vi "ma_Tone estimation subroutine G(f) (FFT input) (CDB).vi"(8 "N (window length)":i32=512, 9 "window":u16(ring) items=["Rectangle"=0, "Hanning"=1, "Hamming"=2, "Blackman-Harris"=3, "Exact Blackman"=4, "Blackman"=5, "Flat Top"=6, "4 Term B-Harris "=7, "7 Term B-Harris"=8, "Low Sidelobe"=9, "Blackman Nuttall"=11, "Triangle"=30, "Bartlett-Hanning"=31, "Bohman"=32, "Parzen"=33, "Welch"=34, "Kaiser"=60, "Dolph-Chebyshev"=61, "Gaussian"=62], 10 "frequency":dbl format="%.5e", 11 "three fingers":T1={"f0"=0.0, "df"=1.0, "spectrum"=[]} {"spectrum" format="%.2f"; "df" format="%.2f"; "f0" format="%.2f"}) -> (1 "phase [degree]":dbl format="%.2f", 2 "Amplitude":dbl format="%.2f", 3 "G(f)":dbl format="%.2e")   [LabVIEW 2020, in "NI_MAPro.lvlib"]
uses:
  NI_MAPro.lvlib
  ma_sml_Spectrum Cluster (complex).ctl
  NI_AALBase.lvlib
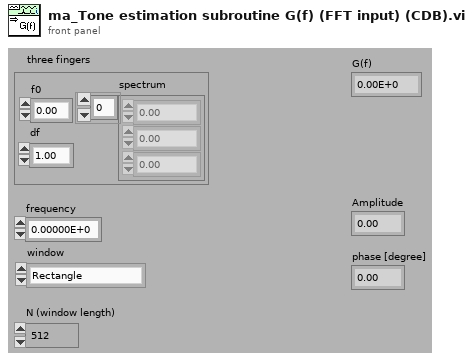
[diagram p1: front panel]
types:
  T1 = typedef "NI_MAPro.lvlib/ma_sml_Spectrum Cluster (complex).ctl" = cluster{"f0":dbl, "df":dbl, "spectrum":cdb[]}
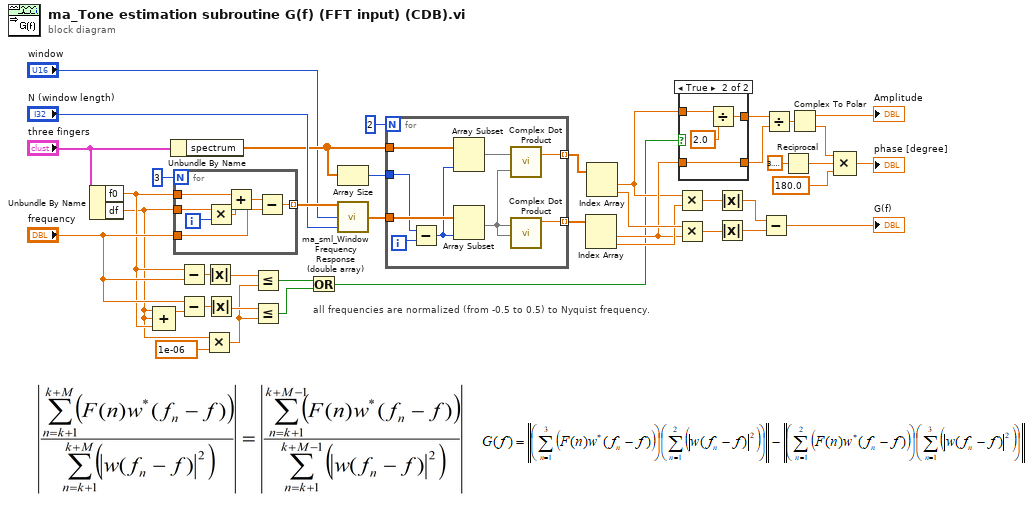
[diagram p0: block diagram]
diagram:
  # "all frequencies are normalized (from -0.5 to 0.5) to Nyquist frequency."
  n1 = Unbundle By Name("three fingers") -> ("f0"=w5:dbl, "df"=w2:dbl)
  n2 = Compound Arithmetic op=ADD(w2, w2, w5) -> (w20:dbl)
  n3 = Unbundle By Name("three fingers") -> ("spectrum"=w6:cdb[])
  n4 = for {
    N: 3 -> [_]
    tunnel: w5 -> [w49]
    tunnel: w2 -> [w46]
    tunnel: "frequency" -> [w44]
    tunnel: [w43] -> w33 mode=indexing
    i -> [w47]
    n5 = Multiply(x=w46, y=w47) -> (x*y=w48:dbl)
    n6 = Add(x=w49, y=w48) -> (x+y=w45:dbl)
    n7 = Subtract(x=w45, y=w44) -> (x-y=w43:dbl)
  }
  n8 = Subtract(x=w5, y="frequency") -> (x-y=w19:dbl)
  n9 = Subtract(x="frequency", y=w20) -> (x-y=w18:dbl)
  n10 = Multiply(x=w2, y=1e-06) -> (x*y=w1:dbl)
  n11 = Absolute Value(x=w19) -> (abs(x)=w17:dbl)
  n12 = Absolute Value(x=w18) -> (abs(x)=w16:dbl)
  n13 = Less Or Equal?(x=w17, y=w1) -> (x <= y?=w15:bool)
  n14 = Less Or Equal?(x=w16, y=w1) -> (x <= y?=w9:bool)
  n15 = Or(x=w15, y=w9) -> (x .or. y?=w8:bool)
  n16 = Array Size(array=w6) -> (size(s)=w26:i32)
  n17 = call "ma_sml_Window Frequency Response (double array).vi"("N (window length)"="N (window length)", "window"="window", "f(normalized)"=w33) -> ("H(f)"=w32:cdb[])
  n18 = for {
    N: 2 -> [_]
    tunnel: w6 -> [w58]
    tunnel: w32 -> [w57]
    tunnel: [w51] -> w30 mode=indexing
    tunnel: [w50] -> w29 mode=indexing
    tunnel: w26 -> [w55]
    i -> [w54]
    n19 = Subtract(x=w55, y=w54) -> (x-y=w56:i32)
    n20 = Array Subset(array=w58, length=w56) -> (w52:cdb[])  [unwired: 1 in]
    n21 = Array Subset(array=w57, length=w56) -> (w53:cdb[])  [unwired: 1 in]
    n22 = call "Complex Dot Product.vi"("Y Vector"=w53, "X Vector"=w52) -> ("X * Y"=w51:cdb)  [unwired: 1 out]
    n23 = call "Complex Dot Product.vi"("Y Vector"=w53, "X Vector"=w53) -> ("X * Y"=w50:cdb)  [unwired: 1 out]
  }
  n24 = Index Array(array=w29) -> (element #1=w14:cdb, element #2=w23:cdb)  [unwired: 2 in]
  n25 = Index Array(array=w30) -> (element #1=w12:cdb, element #2=w24:cdb)  [unwired: 2 in]
  n26 = Multiply(x=w12, y=w23) -> (x*y=w28:cdb)
  n27 = Multiply(x=w24, y=w14) -> (x*y=w27:cdb)
  n28 = case shown="True" w8 {
    tunnel: w14 -> [w60 w62]
    tunnel: [w60 w62] -> w13
    tunnel: w12 -> [w59 w61]
    tunnel: [w59 w64] -> w11
    frame False {
    }
    frame True {
      n29 = Divide(x=w61, y=2.0) -> (x/y=w64:cdb)
    }
  }
  n30 = Absolute Value(x=w28) -> (abs(x)=w41:dbl)
  n31 = Absolute Value(x=w27) -> (abs(x)=w40:dbl)
  n32 = Subtract(x=w41, y=w40) -> (x-y=→"G(f)":dbl)
  n33 = Divide(x=w11, y=w13) -> (x/y=w22:cdb)
  n34 = Reciprocal(x=3.141592653589793) -> (1/x=w37:dbl)
  n35 = Complex To Polar(r * e^(i*theta)=w22) -> (r=→"Amplitude":dbl, theta=w39:dbl)
  n36 = Compound Arithmetic op=MULTIPLY(w39, w37, 180.0 ("Input")) -> (→"phase [degree]":dbl)
